vi "Flatten to String.vi"(8 "error in (no error)":errorcluster, 11 "ISerializable in":refnum<class "ISerializable.lvclass">) -> (0 "error out":errorcluster, 3 "Flattened Class":string)   [LabVIEW 2019, in "Composed Log.lvlib" / "ISerializable.lvclass"]
uses:
  <vilib>/gpm_packages/@cs/event-logger/Source/Composed Log/ISerializable/ISerializable.lvclass
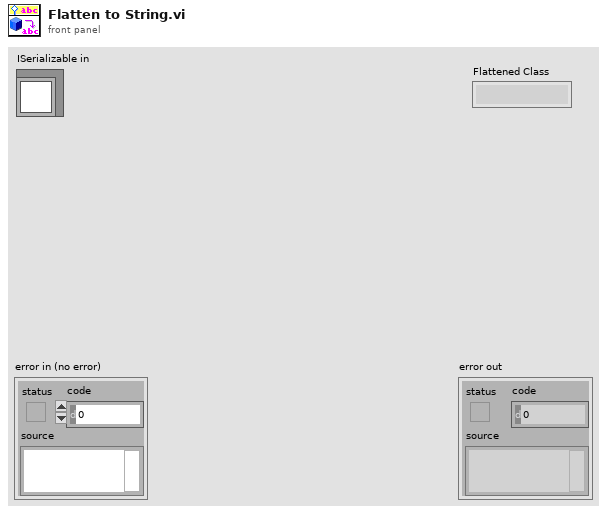
[diagram p1: front panel]
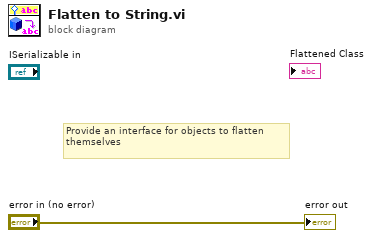
[diagram p0: block diagram]
diagram:
  # "Provide an interface for objects to flatten themselves"
  "error out" <- "error in (no error)"
